vi "Check For Errors.vi"(7 "Mode":T1(ring), 8 "error in (no error)":errorcluster, 11 "LUnit Test Case In":refnum<class "LUnit Test Case.lvclass">) -> (0 "error out":errorcluster, 3 "LUnit Test Case Out":refnum<class "LUnit Test Case.lvclass">)   [LabVIEW 2020, in "LUnit Test Case.lvclass"]
uses:
  LUnit Test Case.lvclass
  LUnit Test Case.lvclass/LUnit Test Case.ctl
  Result Classes/Test Case Result/Test Case Result.lvclass/Test Case Result.ctl
  Result Classes/Method Result/Method Result.lvclass/Method Result.ctl
  Result Classes/Method Result/Public/Read Status.vi
  Result Classes/Method Result/Community/Accessors/Generate Error.vi
  Result Classes/Test Case Result/Test Case Result.lvclass
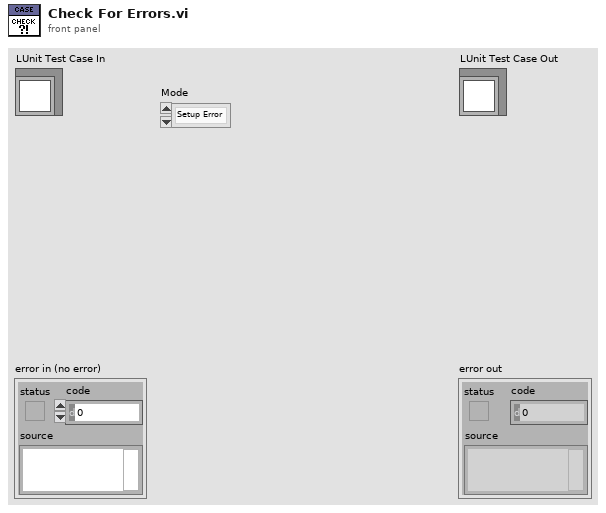
[diagram p1: front panel]
types:
  T1 = enum16{"Setup Error", "Teardown Error", "Broken", "Test Method Error"}
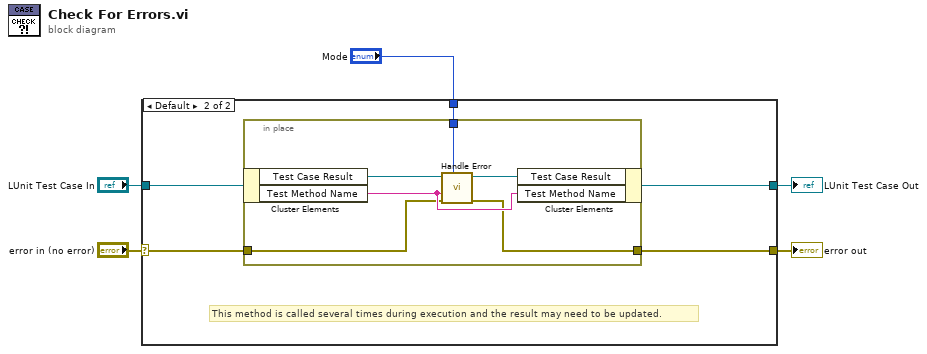
[diagram p0: block diagram]
diagram:
  n1 = case shown="Default" "error in (no error)" {
    selector: "error in (no error)" -> [w7 w11]
    tunnel: [w6 w8] -> w5
    tunnel: "LUnit Test Case In" -> [w6 w12]
    tunnel: [w7 w10] -> w2
    tunnel: "Mode" -> [_ w9]
    frame No Error {
    }
    frame Default {
      # "This method is called several times during execution and the result may need to be updated."
      n2 = in-place {
        in-place-border: w11 -> [w15]
        in-place-border: [w14] -> w10
        in-place-border: w9 -> [w13]
        n3 = in-place-cluster #1(w12) -> ("Test Case Result"=w18:refnum<class "Test Case Result.lvclass">, "Test Method Name"=w16:string)
        n4 = call "Handle Error.vi"("Mode"=w13, "error in (no error)"=w15, "Test Method Name"=w16, "Test Case Result In"=w18) -> ("error out"=w14:errorcluster, "Test Case Result Out"=w17:refnum<class "Test Case Result.lvclass">)  [unwired: 6 in]
        n5 = in-place-cluster #1("Test Case Result"=w17, "Test Method Name"=w16) -> (w8:refnum<class "LUnit Test Case.lvclass">)
      }
    }
  }
  "error out" <- w2
  "LUnit Test Case Out" <- w5
